vi "ARCH_SetPanelOrigin.vi"(8 "error in (no error)":errorcluster caption="错误输入（无错误）", 9 "水平滚动条可见":T1(ring)=enum."Always Off", 10 "origin":T2 caption="原点", 11 "reference":refnum<vi> caption="引用") -> (0 "error out":errorcluster caption="错误输出")   [LabVIEW 2011]
uses:
  <vilib>/Utility/miscctls.llb/LVPointTypeDef.ctl
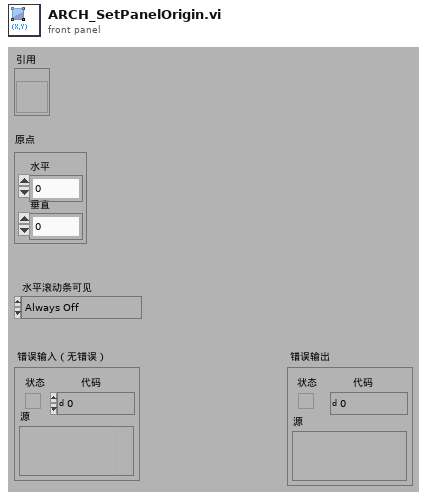
[diagram p1: front panel]
types:
  T1 = enum16{"Always On", "Always Off", "Off While Running"}
  T2 = typedef "LVPointTypeDef.ctl" = cluster{"Horizontal":i16, "Vertical":i16}
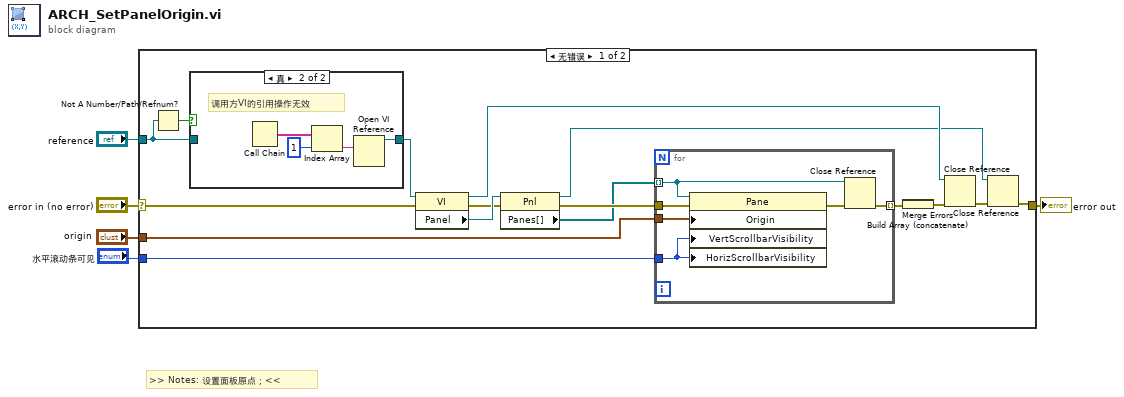
[diagram p0: block diagram]
diagram:
  # ">> Notes: 设置面板原点；<<"
  n1 = case shown="无错误" "error in (no error)" {
    selector: "error in (no error)" -> [w13 w34]
    tunnel: [w9 w34] -> w4
    tunnel: "origin" -> [w14 _]
    tunnel: "reference" -> [w18 _]
    tunnel: "水平滚动条可见" -> [w12 _]
    frame No Error {
      n2 = Not A Number/Path/Refnum?(number/path/refnum=w18) -> (NaN/Path/Refnum?=w19:bool)
      n3 = case shown="真" w19 {
        tunnel: [w29 w30] -> w17
        tunnel: w18 -> [w29 _]
        frame False {
        }
        frame True {
          # "调用方VI的引用操作无效"
          n4 = Call Chain() -> (call chain=w33:string[])
          n5 = Index Array(array=w33, index=1) -> (element=w31:string)
          n6 = Open VI Reference(vi path=w31) -> (vi reference=w30:refnum<vi>)  [unwired: 5 in, 1 out]
        }
      }
      n7 = property on="Property Node" class="VI"(reference=w17, error in=w13) -> (reference out=w20:refnum<vi>, error out=w21:errorcluster, "Panel"=w22:refnum<vi>)
      n8 = property on="Property Node" class="Pnl"(reference=w22, error in=w21) -> (reference out=w15:refnum<vi>, error out=w11:errorcluster, "Panes[]"=w8:refnum<vi>[])
      n9 = for {
        tunnel: w8 -> [w27] mode=indexing
        tunnel: w14 -> [w28]
        tunnel: w11 -> [w25]
        tunnel: [w24] -> w7 mode=indexing
        tunnel: w12 -> [w23]
        n10 = property on="Property Node" class="Pane"(reference=w27, error in=w25, "Origin"=w28, "VertScrollbarVisibility"=w23, "HorizScrollbarVisibility"=w23) -> (error out=w26:errorcluster)  [unwired: 1 out]
        n11 = Close Reference(reference=w27, error in (no error)=w26) -> (error out=w24:errorcluster)
      }
      n12 = Build Array (concatenate)(w7) -> (w6:errorcluster[])
      n13 = Merge Errors(w6) -> (w10:errorcluster)
      n14 = Close Reference(reference=w20, error in (no error)=w10) -> (error out=w16:errorcluster)
      n15 = Close Reference(reference=w15, error in (no error)=w16) -> (error out=w9:errorcluster)
    }
    frame Error {
    }
  }
  "error out" <- w4
